vi "StartMenuPanel.vi"(0 "Play Notifier":refnum<notifier>) -> ()   [LabVIEW 2025]
panel:
  in  "Server Address":string
  in  "Play Button":bool
  in  "Player Name":string
  # "generals.io"
  # "generals.io"
  # "Protect your general. Capture enemy generals."
  # "Player Name"
  # "Server Address"
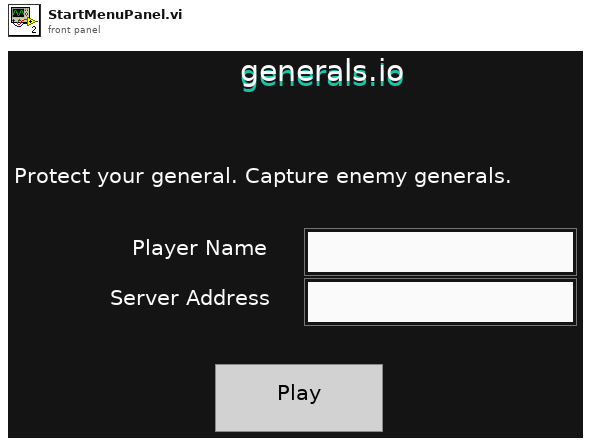
[diagram p1: front panel]
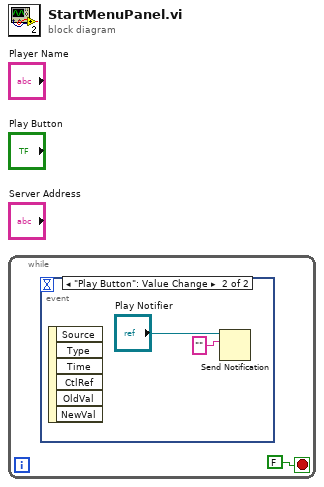
[diagram p0: block diagram]
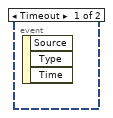
[diagram p2: hidden frame]
diagram:
  n1 = while {
    stop <- FALSE stop-if-true
    n2 = event shown="[1] \"Play Button\": Value Change" {
      selector: _ -> [_ _]
      dyn-events: _ -> [_ _]
      timeout: _ -> [_ _]
      event Timeout {
        n3 = event-data() -> ()  [unwired: 1 in, 3 out]
      }
      event "Play Button": Value Change {
        n4 = event-data() -> ()  [unwired: 1 in, 6 out]
        n5 = Send Notification(notification="", notifier="Play Notifier") -> ()  [unwired: 1 in, 2 out]
      }
    }
  }
